vi "5012 Unexpected Control Data Type.vi"(8 "error in (no error)":errorcluster, 10 "Expecting Scalar?":bool, 11 "Control Name":string) -> (0 "error out":errorcluster)   [LabVIEW 2020, in "MacroAssert.lvlib" / "Custom Errors.lvlib"]
uses:
  Custom Errors.lvlib
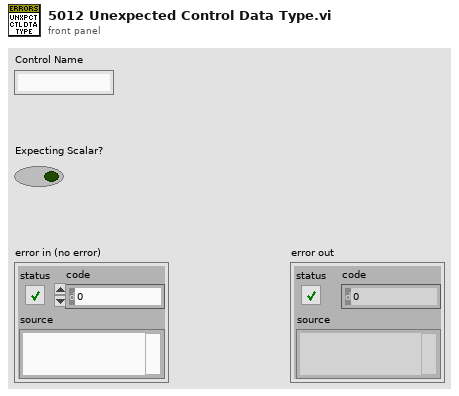
[diagram p1: front panel]
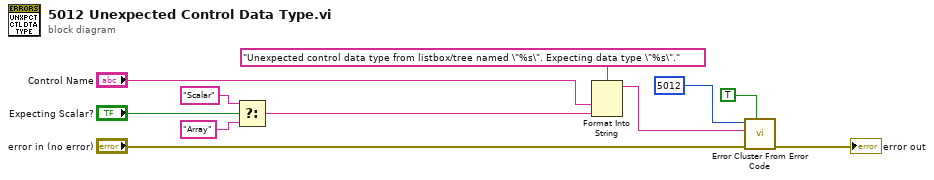
[diagram p0: block diagram]
diagram:
  n1 = Select(t="Scalar", s="Expecting Scalar?", f="Array") -> (s? t:f=w1:string)
  n2 = Format Into String(format string="Unexpected control data type from listbox/tree named \"%s\". Expecting data type \"%s\".", "Control Name", w1) -> (resulting string=w7:string)  [unwired: 2 in, 1 out]
  n3 = call <vilib>:"Error Cluster From Error Code.vi"("show call chain? (False)"=TRUE, "error in (no error)"="error in (no error)", "error message (\"\")"=w7, "error code (0)"=5012) -> ("error out"=→"error out":errorcluster)  [unwired: 5 in]
